vi "tempconfigCI1.vi"(1 "Temp Config in":T1, 2 "command":string) -> (0 "Temp Config out":T1)   [LabVIEW 2015]
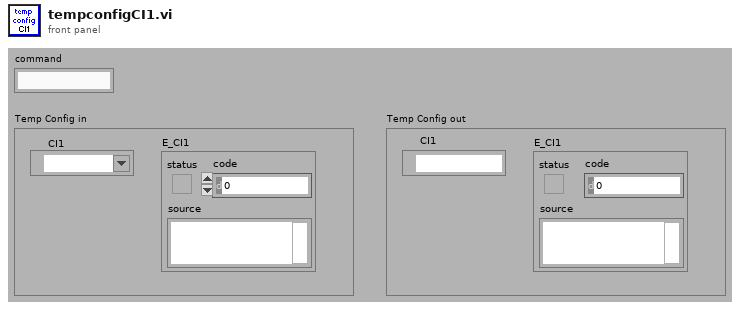
[diagram p1: front panel]
types:
  T1 = cluster{" CI1":refnum<k21>, "E_CI1":errorcluster}
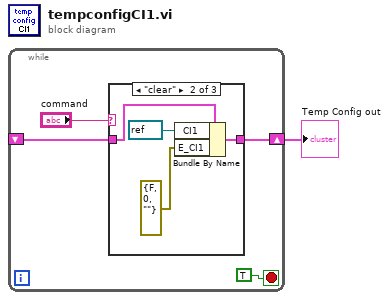
[diagram p0: block diagram]
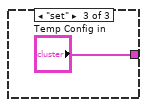
[diagram p3: hidden frame]
diagram:
  n1 = while {
    shift-right: [w3] -> w1
    shift-left: _ -> [w2]
    stop <- TRUE stop-if-true
    n2 = case shown="\"clear\"" "command" {
      tunnel: [w6 w7 "Temp Config in"] -> w3
      tunnel: w2 -> [w6 w10 _]
      frame "get", Default {
      }
      frame "clear" {
        n3 = Bundle By Name(cluster=w10, "CI1"=refnum<k21> refnum ("XY"), "E_CI1"=errorcluster {"status"=FALSE, "code"=0, "source"=""} ("E_AI")) -> (w7:T1)
      }
      frame "set" {
      }
    }
  }
  "Temp Config out" <- w1
